vi "Init File.vi"(6 "Section":string, 7 "create file if necessary (T)":bool=TRUE, 8 "error in (no error)":errorcluster, 10 "configuration file path":path, 11 "Parameter Generic File in":refnum<class "Parameter Generic File.lvclass">) -> (0 "error out":errorcluster, 3 "Parameter Generic File out":refnum<class "Parameter Generic File.lvclass">)   [LabVIEW 2019, in "CD Parameter Manager API.lvlib" / "Parameter Generic File.lvclass"]
uses:
  Parameter Generic File.lvclass
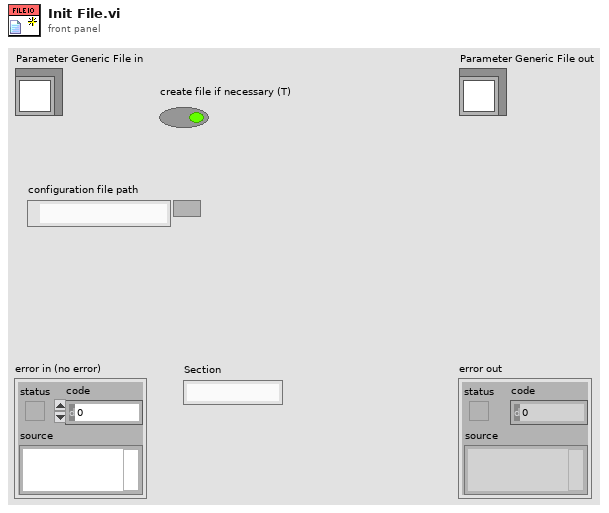
[diagram p1: front panel]
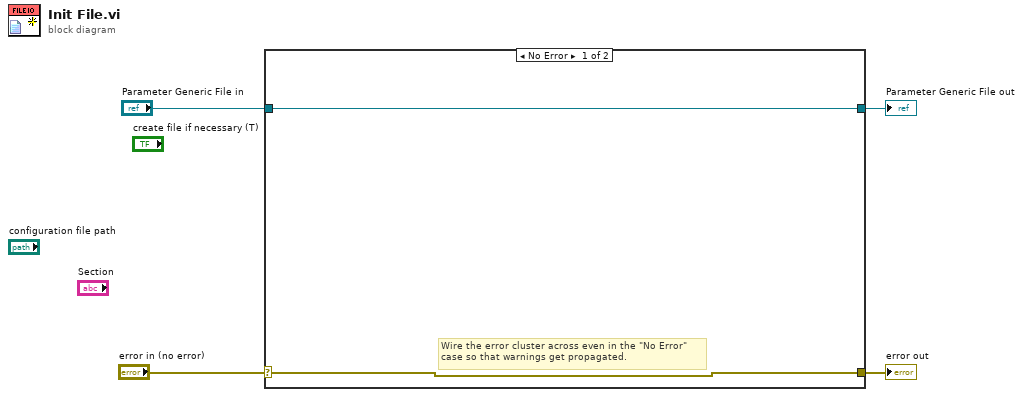
[diagram p0: block diagram]
diagram:
  n1 = case shown="No Error" "error in (no error)" {
    selector: "error in (no error)" -> [w5 w8]
    tunnel: [w5 w8] -> w3
    tunnel: [w6 w7] -> w1
    tunnel: "Parameter Generic File in" -> [w6 w7]
    frame No Error {
      # "Wire the error cluster across even in the \"No Error\"\ncase so that warnings get propagated."
    }
    frame Error {
    }
  }
  "error out" <- w3
  "Parameter Generic File out" <- w1
